vi "Coerce U32 to Variant Intger.vi"(8 "error in (no error)":errorcluster, 9 "Type":T1, 10 "Default in":variant, 11 "U32":u32) -> (0 "error out":errorcluster, 3 "Variant (Data Type) out":variant)   [LabVIEW 2020, in "JSONtext.lvlib"]
uses:
  <vilib>/JDP Science/JSONtext/JSONtext.lvlib
  <vilib>/Utility/Data Type/Type Definitions/Data Type.ctl
  <vilib>/Utility/Data Type/NI_Data Type.lvlib
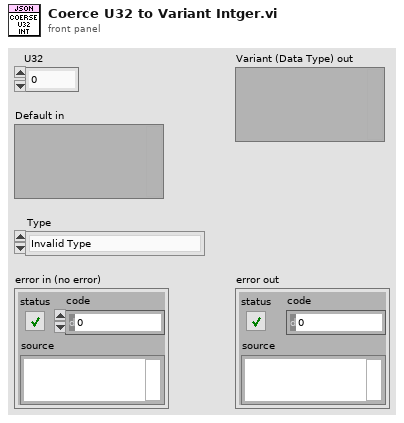
[diagram p1: front panel]
types:
  T1 = typedef "NI_Data Type.lvlib/Data Type.ctl" = enum8{"Invalid Type", "Void", "I8", "I16", "I32", "I64", "U8", "U16", "U32", "U64", "Single Float", "Double Float", "Extended Float", "Single Complex", "Double Complex", "Extended Complex", "Enum U8", "Enum U16", "Enum U32", "Enum U64", "Single Float With Unit", "Double Float With Unit", "Extended Float With Unit", "Single Complex with Unit", "Double Complex with Unit", "Extended Complex with Unit", "Boolean", "String", "Path", "Picture", "Tag", "Array", "Cluster", "Variant", "LV Variant", "Waveform", "Timestamp", "Digital Waveform", "Digital Data", "ExpressData", "Refnum", "External Data", "VI", "Poly VI", "LabVIEW Class Instance", "Fixed Point", "Set Collection", "Map Collection"}
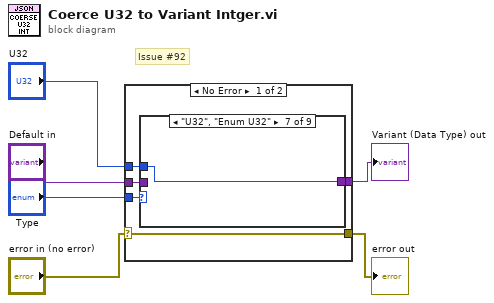
[diagram p0: block diagram]
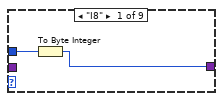
[diagram p2: hidden frame]
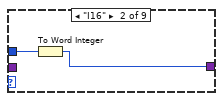
[diagram p3: hidden frame]
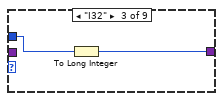
[diagram p4: hidden frame]
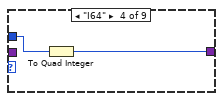
[diagram p5: hidden frame]
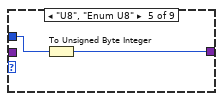
[diagram p6: hidden frame]
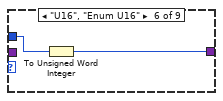
[diagram p7: hidden frame]
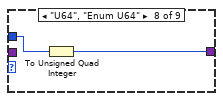
[diagram p8: hidden frame]
diagram:
  # "Issue #92"
  n1 = case shown="No Error" "error in (no error)" {
    selector: "error in (no error)" -> [w7 w28]
    tunnel: "Type" -> [w11 _]
    tunnel: "Default in" -> [w10 w29]
    tunnel: "U32" -> [w9 _]
    tunnel: [w8 w29] -> w4
    tunnel: [w7 w28] -> w6
    frame No Error {
      n2 = case shown="\"U32\", \"Enum U32\"" w11 {
        tunnel: w10 -> [_ _ _ _ _ _ _ _ w27]
        tunnel: [w12 w14 w16 w18 w20 w22 w24 w25 w27] -> w8
        tunnel: w9 -> [w13 w15 w17 w19 w21 w23 w24 w26 _]
        frame "I8" {
          n3 = To Byte Integer(number=w13) -> (8bit integer=w12:i8)
        }
        frame "I16" {
          n4 = To Word Integer(number=w15) -> (16bit integer=w14:i16)
        }
        frame "I32" {
          n5 = To Long Integer(number=w17) -> (32bit integer=w16:i32)
        }
        frame "I64" {
          n6 = To Quad Integer(1:w19) -> (0:w18:i64)
        }
        frame "U8", "Enum U8" {
          n7 = To Unsigned Byte Integer(number=w21) -> (unsigned 8bit integer=w20:u8)
        }
        frame "U16", "Enum U16" {
          n8 = To Unsigned Word Integer(number=w23) -> (unsigned 16bit integer=w22:u16)
        }
        frame "U32", "Enum U32" {
        }
        frame "U64", "Enum U64" {
          n9 = To Unsigned Quad Integer(1:w26) -> (0:w25:u64)
        }
        frame Default {
        }
      }
    }
    frame Error {
    }
  }
  "error out" <- w6
  "Variant (Data Type) out" <- w4
